vi "Write Result.vi"(0 "Charact Result Accessor in":refnum<class "Charact Result Accessor.lvclass">, 5 "Charact Result":variant, 11 "error in":errorcluster) -> (4 "Charact Result Accessor out":refnum<class "Charact Result Accessor.lvclass">, 15 "error out":errorcluster)   [LabVIEW 2023, in "RFFixtureCharact.Public.lvlib" / "Charact Result Accessor.lvclass"]
uses:
  Charact Result Accessor.lvclass
  Charact Result Accessor.lvclass/Charact Result Accessor.ctl
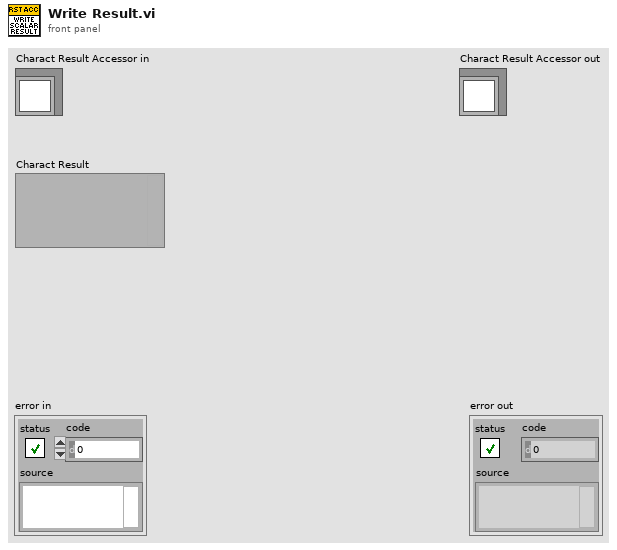
[diagram p1: front panel]
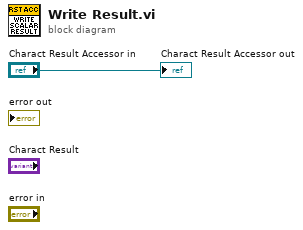
[diagram p0: block diagram]
diagram:
  "Charact Result Accessor out" <- "Charact Result Accessor in"
